vi "checkAmountOfValidImages.vi"(1 "number of required valid images":i32=10, 2 "temp path":path) -> (0 "enough valid images":bool)   [LabVIEW 2012]
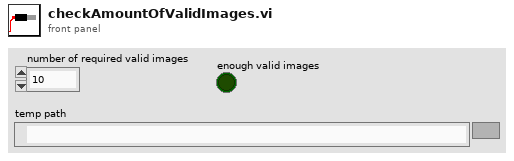
[diagram p1: front panel]
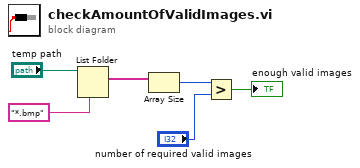
[diagram p0: block diagram]
diagram:
  n1 = List Folder(path="temp path", pattern="*.bmp") -> (filenames=w4:string[])  [unwired: 2 in, 3 out]
  n2 = Array Size(array=w4) -> (size(s)=w3:i32)
  n3 = Greater?(x=w3, y="number of required valid images") -> (0:→"enough valid images":bool)
